vi "MakeSegment Example.vi"() -> ()   [LabVIEW 2010]
uses:
  <vilib>/builds/MDSplus/MDSplus/MDSplus.lvlib
panel:
  out "Overall Waveform":sgl[](graph)
  out "Waveform Graph":dynamicdata(graph)
  in  "stop":bool
  in  "phase":dbl
  in  "amplitude":dbl=5.0
  in  "frequency":dbl=1.1
  in  "Node path":string
  in  "Shot":i32
  in  "Tree Name":string
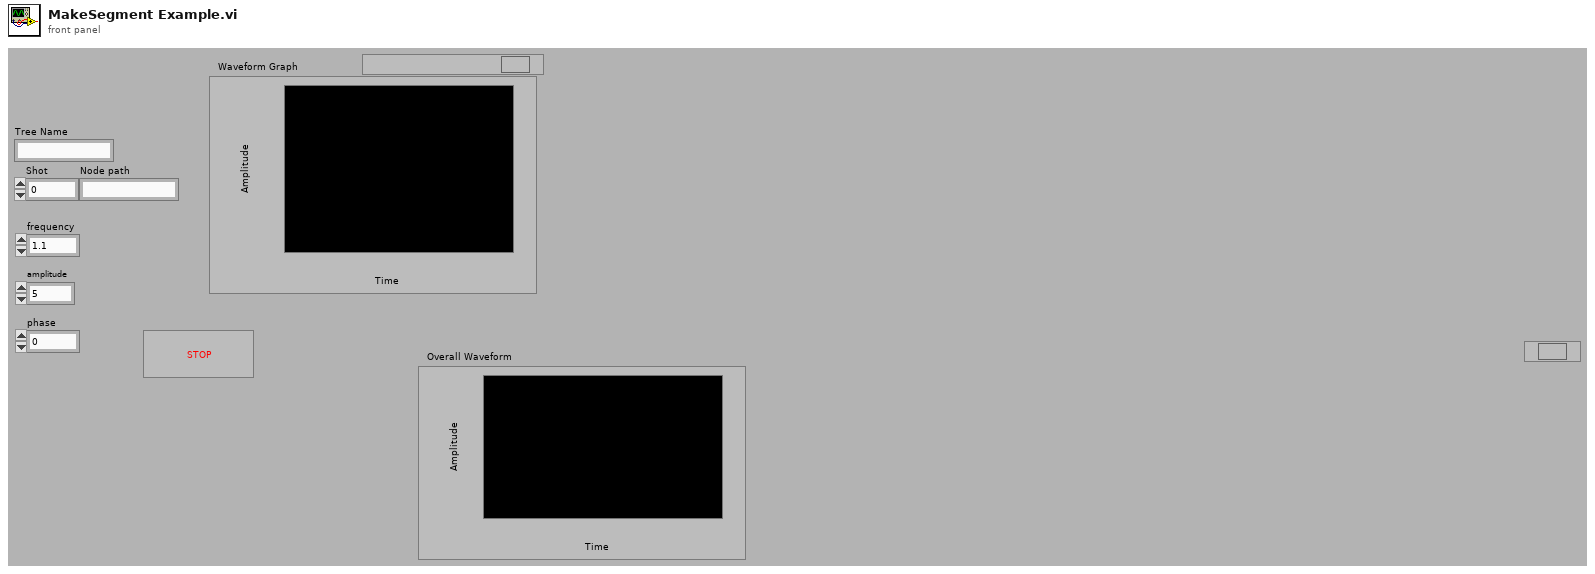
[diagram p1: front panel]
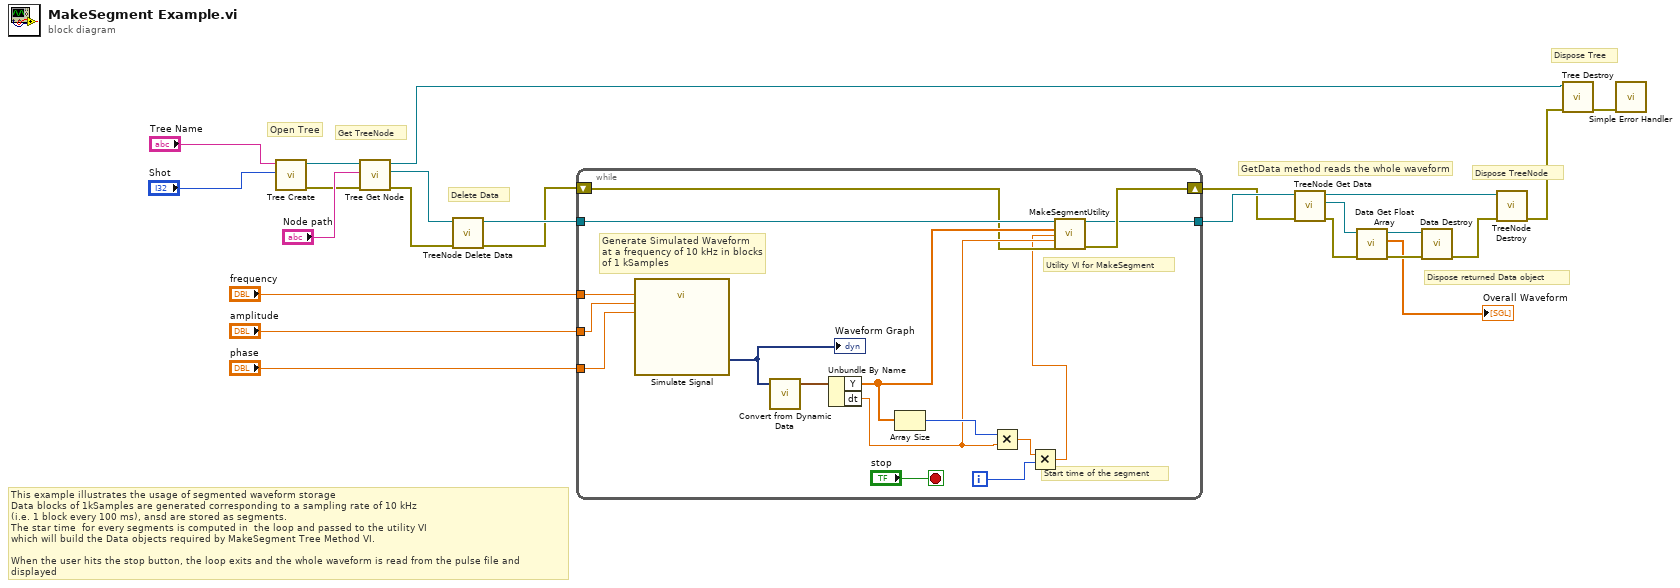
[diagram p0: block diagram]
diagram:
  # "Dispose Tree"
  # "Dispose TreeNode"
  # "GetData method reads the whole waveform"
  # "Dispose returned Data object"
  # "This example illustrates the usage of segmented waveform storage\nData blocks of 1kSamples are generated corresponding to a sampling rate of 10 kHz\n(i.e. 1 block every 100 ms), ansd are stored as segments. \nThe star time  for every segments is computed in  the loop and passed to the utility VI\nwhich will build the Data objects required by MakeSegment Tree Method VI. \n\nWhen the user hits the stop button, the loop exits and the whole waveform is read from the pulse file and displayed"
  # "Delete Data"
  # "Get TreeNode"
  # "Open Tree"
  n1 = call <vilib>:"Tree Create.vi"("Shot"="Shot", "Name"="Tree Name") -> ("error out"=w20:errorcluster, "Tree DVR out"=w22:refnum<data-value>)  [unwired: 8 in]
  n2 = call <vilib>:"Tree Get Node.vi"("error in (no error)"=w20, "Path"="Node path", "Tree DVR in"=w22) -> ("error out"=w2:errorcluster, "Node out"=w3:refnum<data-value>, "Tree DVR out"=w5:refnum<data-value>)  [unwired: 6 in]
  n3 = call <vilib>:"TreeNode Delete Data.vi"("error in (no error)"=w2, "TreeNode DVR in"=w3) -> ("error out"=w1:errorcluster, "TreeNode DVR out"=w4:refnum<data-value>)  [unwired: 8 in]
  n4 = while {
    tunnel: "frequency" -> [w39]
    tunnel: "amplitude" -> [w38]
    tunnel: "phase" -> [w37]
    shift-right: [w27] -> w6
    shift-left: w1 -> [w28]
    tunnel: w4 -> [w35]
    tunnel: [w26] -> w7
    i -> [w30]
    stop <- "stop" stop-if-true
    # "Utility VI for MakeSegment"
    # "Generate Simulated Waveform\nat a frequency of 10 kHz in blocks\nof 1 kSamples"
    # "Start time of the segment"
    n5 = call "Simulate Signal"("Frequency"=w39, "Amplitude"=w38, "Phase"=w37) -> ("Sine with Uniform Noise"=w36:dynamicdata)  [unwired: 11 in, 1 out]
    "Waveform Graph" <- w36
    n6 = call "Convert from Dynamic Data"("Dynamic Data Type"=w36) -> ("Waveform"=w34:waveform(dbl))  [unwired: 3 in]
    n7 = Unbundle By Name(w34) -> ("Y"=w33:dbl[], "dt"=w29:dbl)
    n8 = Array Size(array=w33) -> (size(s)=w32:i32)
    n9 = Multiply(x=w32, y=w29) -> (x*y=w31:dbl)
    n10 = Multiply(x=w31, y=w30) -> (x*y=w25:dbl)
    n11 = call <vilib>:"MakeSegmentUtility.vi"("TreeNode DVR in"=w35, "DBL Array"=w33, "Start time"=w25, "dt"=w29, "error in (no error)"=w28) -> ("TreeNode DVRout"=w26:refnum<data-value>, "error out"=w27:errorcluster)  [unwired: 9 in]
  }
  n12 = call <vilib>:"TreeNode Get Data.vi"("error in (no error)"=w6, "TreeNode DVR in"=w7) -> ("error out"=w12:errorcluster, "Data out"=w13:refnum<data-value>, "TreeNode DVR out"=w14:refnum<data-value>)  [unwired: 7 in]
  n13 = call <vilib>:"Data Get Float Array.vi"("error in (no error)"=w12, "Data DVR in"=w13) -> ("error out"=w11:errorcluster, "SGL array out"=→"Overall Waveform":sgl[], "Data DVR out"=w10:refnum<data-value>)  [unwired: 6 in, 1 out]
  n14 = call <vilib>:"Data Destroy.vi"("error in (no error)"=w11, "Data DVR in"=w10) -> ("error out"=w9:errorcluster)  [unwired: 9 in]
  n15 = call <vilib>:"TreeNode Destroy.vi"("error in (no error)"=w9, "TreeNode DVR in"=w14) -> ("error out"=w15:errorcluster)  [unwired: 9 in]
  n16 = call <vilib>:"Tree Destroy.vi"("error in (no error)"=w15, "Tree DVR in"=w5) -> ("error out"=w16:errorcluster)  [unwired: 9 in]
  n17 = call <vilib>:"Simple Error Handler.vi"("error in (no error)"=w16) -> ()  [unwired: 4 in, 5 out]
